vi "글꼴설정.vi"() -> ()   [LabVIEW 2014]
uses:
  System.Windows.Forms
  System.Drawing
panel:
  out "Name":string
  out "Size":sgl
  out "Color":u32(colorbox) caption="색"
  out "에러 출력":errorcluster
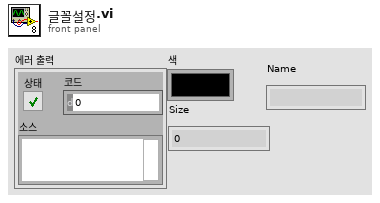
[diagram p1: front panel]
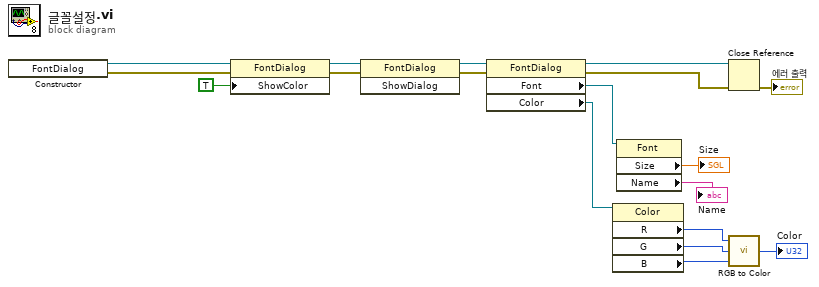
[diagram p0: block diagram]
diagram:
  n1 = constructor class="FontDialog"() -> (reference out=w18:refnum<k24>, error out=w17:errorcluster)  [unwired: 3 in, 1 out]
  n2 = property class="FontDialog"(reference=w18, error in=w17, "ShowColor"=TRUE) -> (reference out=w16:refnum<k24>, error out=w15:errorcluster)
  n3 = invoke class="FontDialog" method="ShowDialog"(reference=w16, error in=w15) -> (reference out=w10:refnum<k24>, error out=w9:errorcluster)  [unwired: 1 in, 1 out]
  n4 = property class="FontDialog"(reference=w10, error in=w9) -> (reference out=w12:refnum<k24>, error out=w11:errorcluster, "Font"=w8:refnum<k24>, "Color"=w7:refnum<k24>)
  n5 = property class="Color"(reference=w7) -> ("R"=w5:u8, "G"=w6:u8, "B"=w4:u8)  [unwired: 1 in, 2 out]
  n6 = property class="Font"(reference=w8) -> ("Size"=→"Size":sgl, "Name"=→"Name":string)  [unwired: 1 in, 2 out]
  n7 = Close Reference(reference=w12, error in (no error)=w11) -> (error out=→"에러 출력":errorcluster)
  n8 = call <vilib>:"RGB to Color.vi"("B"=w4, "G"=w6, "R"=w5) -> ("Color"=→"Color":u32)
